vi "FRCts20_WebMethods_Teams_GET.vi"(7 "httpRequestID":u32, 8 "View":string, 9 "select-choice-software":string, 10 "select-choice-location":string) -> ()   [LabVIEW 2014, in "FRCts20_WebMethods.lvlib"]
uses:
  FRCts20_WebMethods.lvlib
  ESP Engine/source/VI Source/FRCts20_EspEngine.lvlib
  Backend/source/VI Source/FRCts20_Backend_API/FRCts20_Backend_API.lvlib
  Backend/source/VI Source/FRCts20_Backend_API/FRCts20_Backend_API_Event.vi
  Backend/source/VI Source/FRCts20_Backend_API/FRCts20_Backend_API_SW.ctl
  Backend/source/VI Source/FRCts20_Backend_API/FRCts20_Backend_API_Event.ctl
  Backend/source/VI Source/FRCts20_Backend_API/FRCts20_Backend_API_Command_Event.ctl
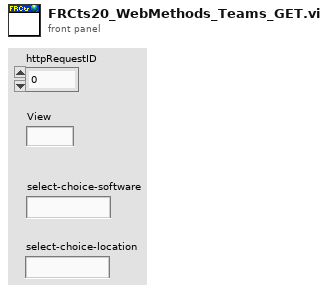
[diagram p1: front panel]
types:
  T1 = typedef "FRCts20_EspEngine.lvlib/FRCts20_EspEngine_SearchBrowser.ctl" = cluster{"Event":cluster{"Event Index":u32, "Event Name":string, "Start Time":timestamp, "End Time":timestamp, "OpenIssues":u8, "IsLive":bool}[], "select-choice-software":string, "select-choice-location":string}
  T2 = typedef "FRCts20_Backend_API.lvlib/FRCts20_Backend_API_Command_Event.ctl" = string
  T3 = typedef "FRCts20_Backend_API.lvlib/FRCts20_Backend_API_Event.ctl" = cluster{"Event Index":u32, "Name":string, "Start Time":timestamp, "End Time":timestamp, "Teams":cluster{"Team Index":u32, "Team Number":u32, "Requests":cluster{"Request Number":u32, "Description":string}[], "Has Open Issue":bool}[], "SWType":T4, "APIReturn":string}
  T4 = typedef "FRCts20_Backend_API.lvlib/FRCts20_Backend_API_SW.ctl" = string
  T5 = typedef "FRCts20_EspEngine.lvlib/FRCts20_EspEngine_Event.ctl" = cluster{"Single Event":T6, "EventOpenIssueCount":i16, "Requests":cluster{"RequestId":i32, "Request Description":string, "Team Number":i32}[], "ClosedRequests":cluster{"RequestId":i32, "Request Description":string, "Team Number":i32}[], "NotFoundStatus":bool}
  T6 = typedef "FRCts20_WebMethods.lvlib/FRCts20_WebMethods_ctl_singleEvent.ctl" = cluster{"Team":T7[], "Issue Count":i32, "Location":string, "Start Date ":timestamp}
  T7 = typedef "FRCts20_WebMethods.lvlib/FRCts20_WebMethods_ctl_teamIdentifier.ctl" = cluster{"Team Nickname":string, "Team Number ":u32, "UniqueId":u32}
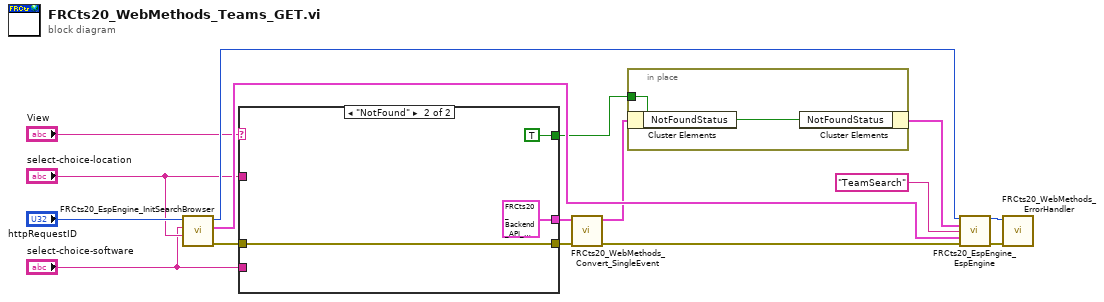
[diagram p0: block diagram]
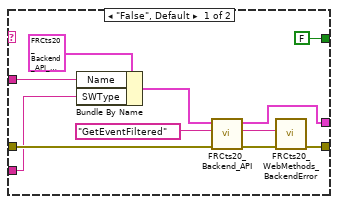
[diagram p2: hidden frame]
diagram:
  n1 = call "FRCts20_EspEngine_InitSearchBrowser.vi"("select-choice-location"="select-choice-location", "select-choice-software"="select-choice-software", "httpRequestID"="httpRequestID") -> ("error out"=w8:errorcluster, "SearchBrowser"=w11:T1, "httpRequestID out"=w12:u32)  [unwired: 6 in]
  n2 = case shown="\"NotFound\"" "View" {
    tunnel: [FALSE TRUE] -> w9
    tunnel: [w24 w29] -> w6
    tunnel: w8 -> [w23 w29]
    tunnel: [w22 T3 {"Event Index"=0, "Name"="", "Start Time"=timestamp(0 s since 1904-01-01), "End Time"=timestamp(0 s since 1904-01-01), "Teams"=[], "SWType"="", "APIReturn"=""} ("Event Out")] -> w2
    tunnel: "select-choice-location" -> [w20 _]
    tunnel: "select-choice-software" -> [w19 _]
    frame "False", Default {
      n3 = Bundle By Name(cluster=T3 {"Event Index"=0, "Name"="", "Start Time"=timestamp(0 s since 1904-01-01), "End Time"=timestamp(0 s since 1904-01-01), "Teams"=[], "SWType"="", "APIReturn"=""} ("Event In"), "Name"=w20, "SWType"=w19) -> (w18:T3)
      n4 = call-poly "FRCts20_Backend_API.vi"("error in (no error)"=w23, "Command"=T2 "GetEventFiltered", "Event In"=w18) -> ("error out"=w26:errorcluster, "Status"=w25:string, "Event Out"=w22:T3)  [unwired: 6 in]
      n5 = call "FRCts20_WebMethods_BackendError.vi"("error in (no error)"=w26, "Status"=w25) -> ("error out"=w24:errorcluster)  [unwired: 8 in, 1 out]
    }
    frame "NotFound" {
    }
  }
  n6 = call "FRCts20_WebMethods_Convert_SingleEvent.vi"("error in (no error)"=w6, "Event Out"=w2) -> ("error out"=w5:errorcluster, "Event"=w1:T5)  [unwired: 8 in]
  n7 = in-place {
    in-place-border: w9 -> [w31]
    n8 = in-place-cluster #1(w1) -> ()  [unwired: 1 out]
    n9 = in-place-cluster #1("NotFoundStatus"=w31) -> (w13:T5)
  }
  n10 = call "FRCts20_EspEngine_EspEngine.vi"("httpRequestID"=w12, "Cluster"=w13, "Page"="TeamSearch", "SearchBrowser"=w11, "error in (no error)"=w5) -> ("httpRequestID out"=w14:u32, "error out"=w15:errorcluster)  [unwired: 9 in]
  n11 = call "FRCts20_WebMethods_ErrorHandler.vi"("error in"=w15, "httpRequestID"=w14) -> ()  [unwired: 9 in, 1 out]
